vi "TrimScanParams.vi"(8 "Parameters to change":i32, 9 "Step Sizes":dbl[](array[numeric]), 10 "Final Values":dbl[](array[numeric]), 11 "Initial Values":dbl[](array[numeric])) -> (1 "Step Sizes Out":dbl[](array[numeric]), 2 "Final Values Out":dbl[](array[numeric]), 3 "Initial Values Out":dbl[](array[numeric]))   [LabVIEW 2016]
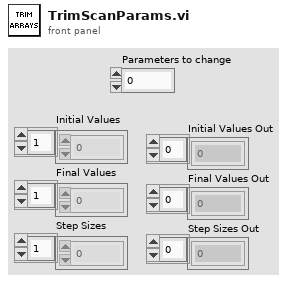
[diagram p1: front panel]
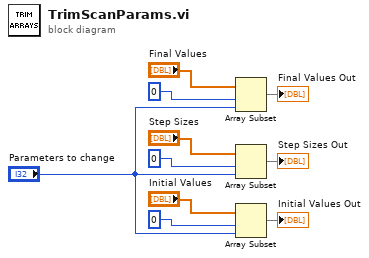
[diagram p0: block diagram]
diagram:
  n1 = Array Subset(array="Final Values", index=0, length="Parameters to change") -> (→"Final Values Out":dbl[])
  n2 = Array Subset(array="Step Sizes", index=0, length="Parameters to change") -> (→"Step Sizes Out":dbl[])
  n3 = Array Subset(array="Initial Values", index=0, length="Parameters to change") -> (→"Initial Values Out":dbl[])
